vi "ParametresCommande.vi"(4 "Diametre Galet Codeur":dbl, 5 "Ressolution Codeur":dbl, 6 "Diametre Plateau":dbl, 7 "Accel":dbl, 8 "Decel Max":dbl, 9 "Accel Max":dbl, 10 "Vitesse Max":dbl, 11 "Decel":dbl) -> ()   [LabVIEW 2015]
uses:
  Variable globale.vi
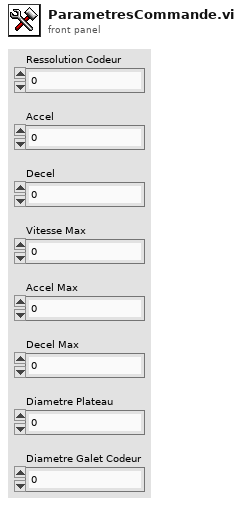
[diagram p1: front panel]
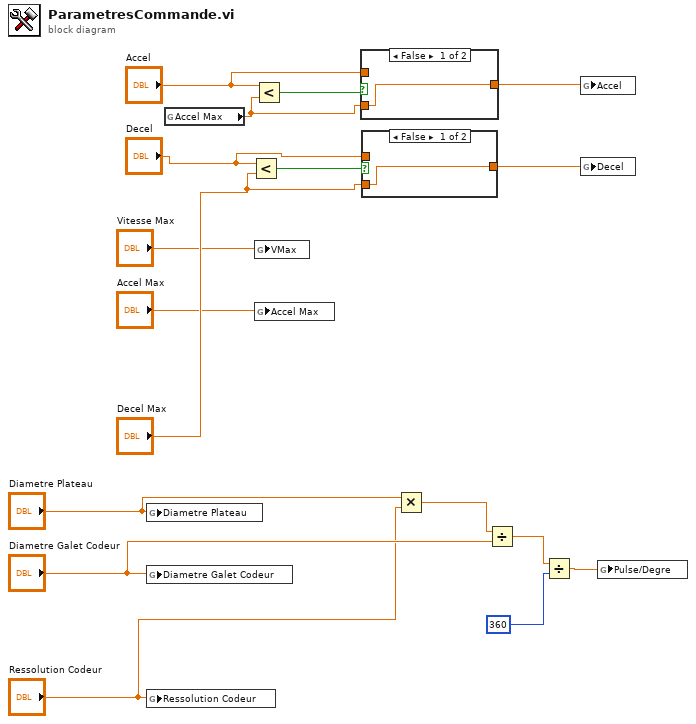
[diagram p0: block diagram]
diagram:
  n1 = global write "Variable globale.vi" "Diametre Plateau"("Diametre Plateau") -> ()
  n2 = global write "Variable globale.vi" "Diametre Galet Codeur"("Diametre Galet Codeur") -> ()
  n3 = global write "Variable globale.vi" "Ressolution Codeur"("Ressolution Codeur") -> ()
  n4 = global read "Variable globale.vi" "Accel Max"() -> (w12:dbl)
  n5 = Less?(x="Decel", y="Decel Max") -> (x < y?=w14:bool)
  n6 = Less?(x="Accel", y=w12) -> (x < y?=w10:bool)
  n7 = global write "Variable globale.vi" "VMax"("Vitesse Max") -> ()
  n8 = global write "Variable globale.vi" "Accel Max"("Accel Max") -> ()
  n9 = case shown="False" w10 {
    tunnel: "Accel" -> [_ w19]
    tunnel: w12 -> [w18 _]
    tunnel: [w18 w19] -> w13
    frame False {
    }
    frame True {
    }
  }
  n10 = case shown="False" w14 {
    tunnel: "Decel" -> [_ w21]
    tunnel: "Decel Max" -> [w20 _]
    tunnel: [w20 w21] -> w16
    frame False {
    }
    frame True {
    }
  }
  n11 = Multiply(x="Diametre Plateau", y="Ressolution Codeur") -> (x*y=w5:dbl)
  n12 = Divide(x=w5, y="Diametre Galet Codeur") -> (x/y=w7:dbl)
  n13 = Divide(x=w7, y=360) -> (x/y=w9:dbl)
  n14 = global write "Variable globale.vi" "Accel"(w13) -> ()
  n15 = global write "Variable globale.vi" "Decel"(w16) -> ()
  n16 = global write "Variable globale.vi" "Pulse/Degre"(w9) -> ()
